vi "data_read.vi"() -> ()   [LabVIEW 2013]
panel:
  out "Waveform Graph 3":sgl[](graph)
  out "new data":cluster{sgl[], sgl[]}(graph)
  in  "Y 3":i32
  in  "X 3":i32
  out "Waveform Graph 2":sgl[](graph)
  out "total data":cluster{sgl[], sgl[]}(graph)
  in  "Y 2":i32
  in  "X 2":i32
  in  "add path":path
  out "Waveform Graph":sgl[](graph)
  out "XY Graph":cluster{sgl[], sgl[]}(graph)
  in  "Y":i32
  in  "X":i32
  in  "error in":errorcluster
  in  "Path":path
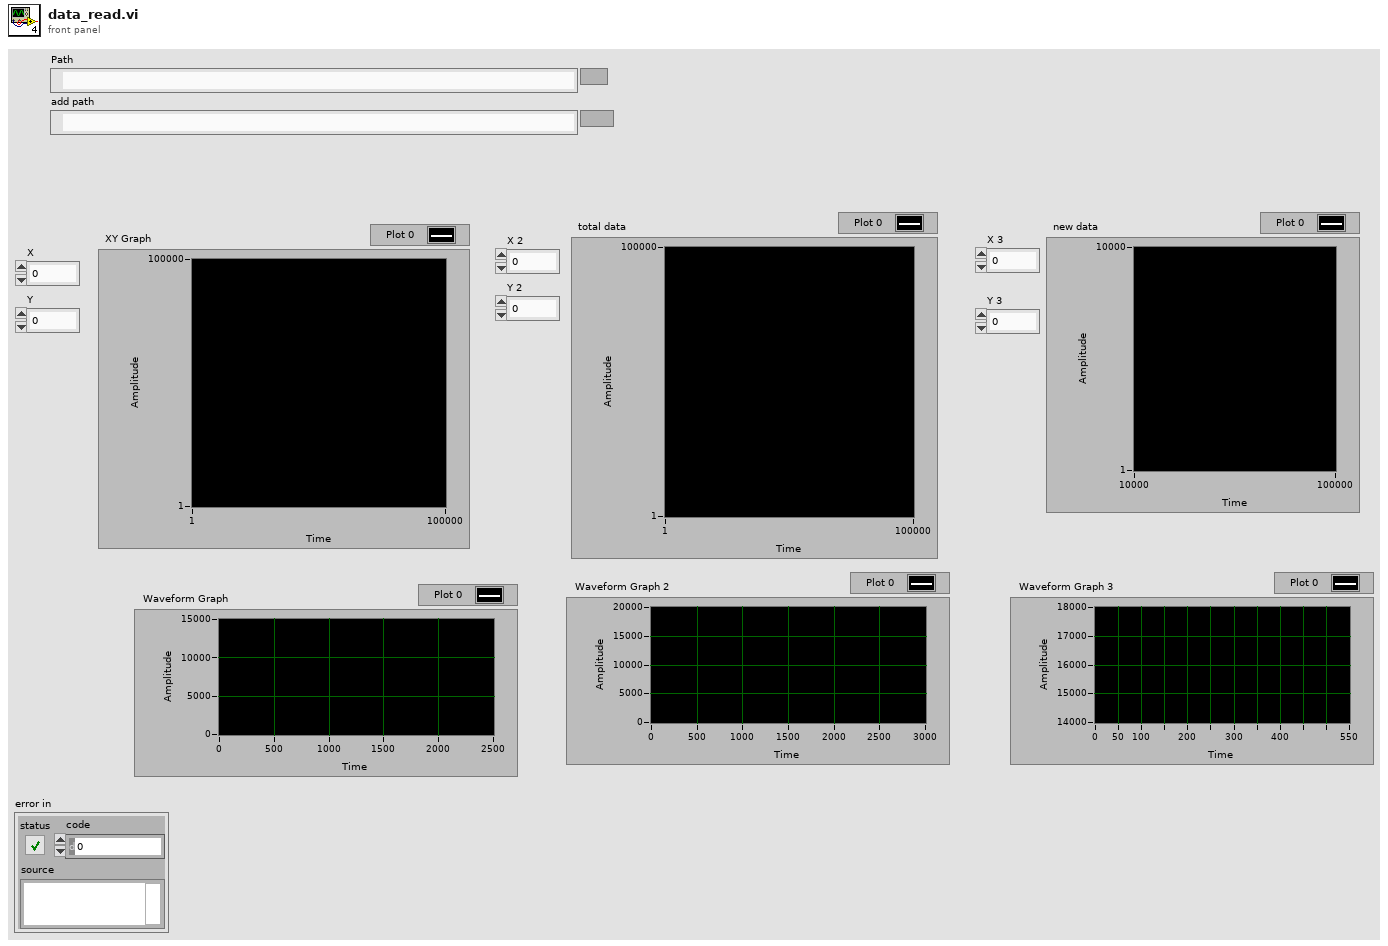
[diagram p1: front panel]
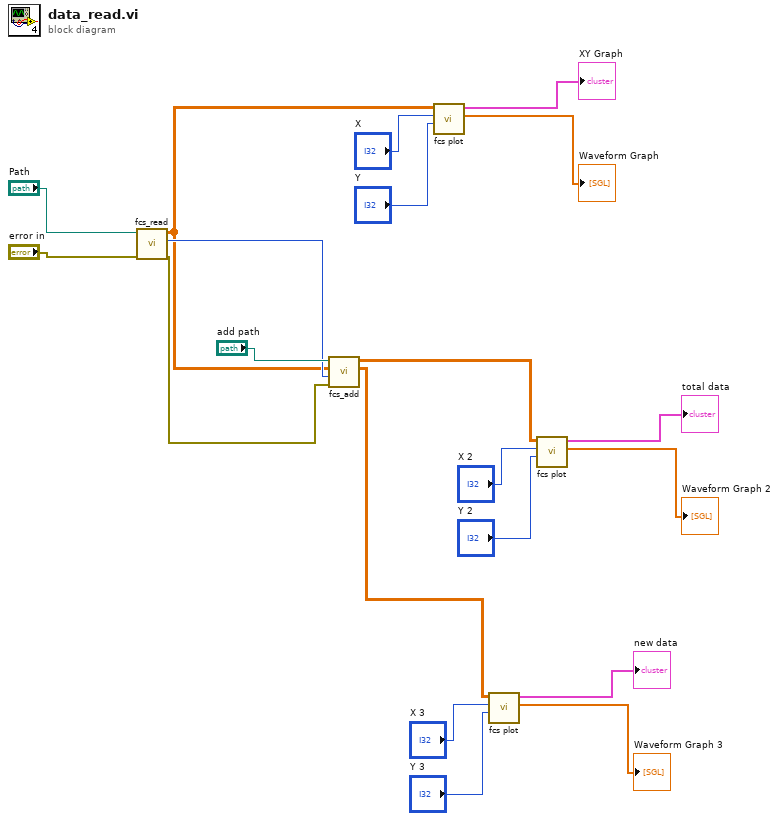
[diagram p0: block diagram]
diagram:
  n1 = call "fcs_read.vi"("error in (no error)"="error in", "Path"="Path") -> ("error out"=w14:errorcluster, "byte offset"=w12:i64, "Array"=w11:sgl[][])  [unwired: 6 in, 1 out]
  n2 = call "fcs_add.vi"("error in (no error)"=w14, "byte offset in"=w12, "Array in"=w11, "Path in"="add path") -> ("new data"=w1:sgl[][], "total data"=w6:sgl[][])  [unwired: 4 in, 2 out]
  n3 = call "fcs plot.vi"("par2"="Y", "par1"="X", "Array in"=w11) -> ("par1 plot"=→"Waveform Graph":sgl[], "xy plot"=→"XY Graph":cluster{"Array":sgl[], "Array":sgl[]})  [unwired: 7 in]
  n4 = call "fcs plot.vi"("par2"="Y 3", "par1"="X 3", "Array in"=w1) -> ("par1 plot"=→"Waveform Graph 3":sgl[], "xy plot"=→"new data":cluster{"Array":sgl[], "Array":sgl[]})  [unwired: 7 in]
  n5 = call "fcs plot.vi"("par2"="Y 2", "par1"="X 2", "Array in"=w6) -> ("par1 plot"=→"Waveform Graph 2":sgl[], "xy plot"=→"total data":cluster{"Array":sgl[], "Array":sgl[]})  [unwired: 7 in]
